vi "GainNumber2Value.vi"(10 "Gain permitted values":u32[](array[numeric])=[0, 16, 32, 48, 64, 80, 96, 112, 128, 144, 160, 176, 192, 208, 224, 240, 256, 288, 320, 352, 384, 416, 448, 480, 512, 544, 576, 608, 640, 672, 704, 736, 768, 832, 896, 960, 1024, 1088, 1152, 1216, 1280, 1344, 1408, 1472, 1536, 1600, 1664, 1728], 11 "Numeric":dbl) -> (3 "Value":u32)   [LabVIEW 2015]
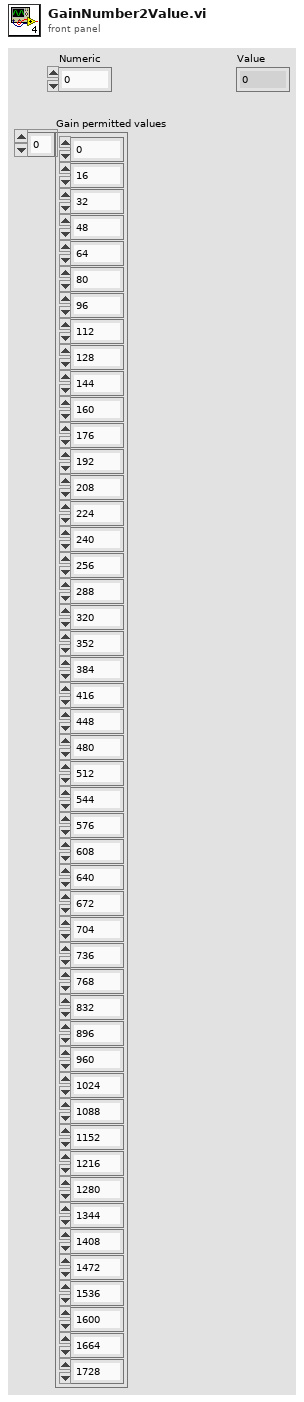
[diagram p1: front panel]
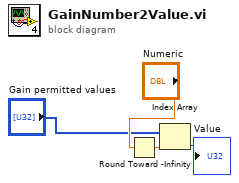
[diagram p0: block diagram]
diagram:
  n1 = Round Toward -Infinity(1:"Numeric") -> (0:w2:dbl)
  n2 = Index Array(array="Gain permitted values", index=w2) -> (element=→"Value":u32)
